vi "Clean.vi"(0 "Compound_Installer in":refnum<class "Compound_Installer.lvclass">) -> (4 "Compound_Installer out":refnum<class "Compound_Installer.lvclass">)   [LabVIEW 2017, in "CL_G3_VIComponentBuilder.lvlib" / "Compound_Installer.lvclass"]
doc: "Removes this export from the build machine."
uses:
  Compound_Installer.lvclass
  C:/Tool Chain Support/Software Module Builder/Source/Exports/Exports/Export.lvclass
  Exports/Export.lvclass/Export.ctl
  Compound_Installer.lvclass/Compound_Installer.ctl
  Exports/Accessors/Write Export Operation Errors.vi
  Exports/Accessors/Read Component Export Dir.vi
  Exports/Accessors/Read Export Operation Errors.vi
  Accessors/Read Sub Export Build Order.vi
  Exports/Export.lvclass
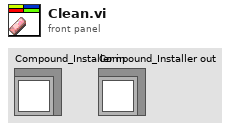
[diagram p1: front panel]
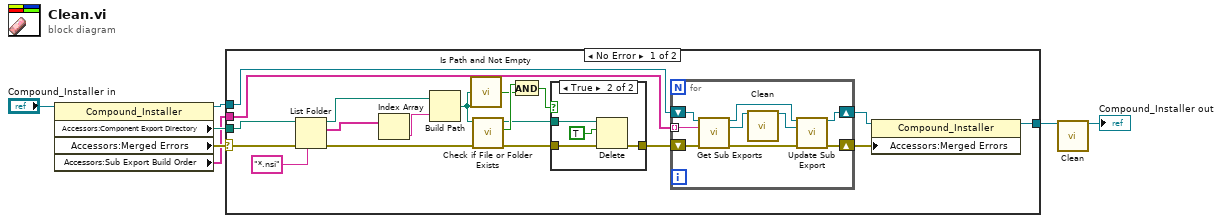
[diagram p0: block diagram]
diagram:
  n1 = property class="Compound_Installer"(reference="Compound_Installer in") -> (reference out=w6:refnum<class "Compound_Installer.lvclass">, "Accessors:Component Export Directory"=w5:path, "Accessors:Merged Errors"=w7:errorcluster, "Accessors:Sub Export Build Order"=w1:string[])  [unwired: 1 in, 1 out]
  n2 = case shown="No Error" w7 {
    selector: w7 -> [w23 _]
    tunnel: w6 -> [w12 w41]
    tunnel: [w26 w41] -> w3
    tunnel: w5 -> [w25 _]
    tunnel: w1 -> [w13 _]
    frame No Error {
      n3 = List Folder(path=w25, pattern="*.nsi", error in=w23) -> (path out=w8:path, filenames=w22:string[], error out=w18:errorcluster)  [unwired: 1 in, 1 out]
      n4 = Index Array(array=w22) -> (element=w21:string)  [unwired: 1 in]
      n5 = Build Path(base path=w8, name or relative path=w21) -> (appended path=w16:path)
      n6 = call <vilib>:"Is Path and Not Empty.vi"("path"=w16) -> ("Is Path and Not Empty?"=w14:bool)  [unwired: 4 in]
      n7 = call <vilib>:"Check if File or Folder Exists.vi"("error in (no error)"=w18, "path"=w16) -> ("error out"=w17:errorcluster, "file or folder exists?"=w20:bool, "dup path"=w19:path)  [unwired: 7 in]
      n8 = And(x=w20, y=w14) -> (x .and. y?=w15:bool)
      n9 = case shown="True" w15 {
        tunnel: [w36 w39] -> w10
        tunnel: w19 -> [_ w38]
        tunnel: w17 -> [w36 w37]
        frame False {
        }
        frame True {
          n10 = Delete(path (use dialog)=w38, entire hierarchy (F)=TRUE, error in=w37) -> (error out=w39:errorcluster)  [unwired: 2 in, 2 out]
        }
      }
      n11 = for {
        tunnel: w13 -> [w34] mode=indexing
        shift-right: [w30] -> w11
        shift-left: w12 -> [w35]
        shift-right: [w27] -> w9
        shift-left: w10 -> [w29]
        n12 = call-dynamic "Get Sub Exports.vi"("NSIS_Installer in"=w35, "Sub Installer Name"=w34, "error in (no error)"=w29) -> ("NSIS_Installer out"=w32:refnum<class "Compound_Installer.lvclass">, "Export"=w33:refnum<class "Export.lvclass">, "error out"=w28:errorcluster)  [unwired: 9 in, 1 out]
        n13 = call-dynamic "Clean.vi"("Export in"=w33) -> ("Export out"=w31:refnum<class "Export.lvclass">)  [unwired: 14 in]
        n14 = call-dynamic "Update Sub Export.vi"("NSIS_Installer in"=w32, "Sub Export"=w31, "error in (no error)"=w28) -> ("NSIS_Installer out"=w30:refnum<class "Compound_Installer.lvclass">, "error out"=w27:errorcluster)  [unwired: 11 in]
      }
      n15 = property class="Compound_Installer"(reference=w11, "Accessors:Merged Errors"=w9) -> (reference out=w26:refnum<class "Compound_Installer.lvclass">)  [unwired: 1 in, 1 out]
    }
    frame Error {
    }
  }
  n16 = call-parent "Clean.vi"("Export in"=w3) -> ("Export out"=→"Compound_Installer out":refnum<class "Compound_Installer.lvclass">)  [unwired: 14 in]
